vi "日期键盘.vi"(11 "原值":string) -> (3 "x+y":string)   [LabVIEW 2016]
uses:
  <vilib>/Utility/miscctls.llb/LVPointTypeDef.ctl
panel:
  in  "日":string(combo)="01"
  in  "月":string(combo)="01"
  in  "年":string(combo)="2000"
  in  "取消按钮":bool
  in  "停止":bool
  # "年"
  # "月"
  # "日"
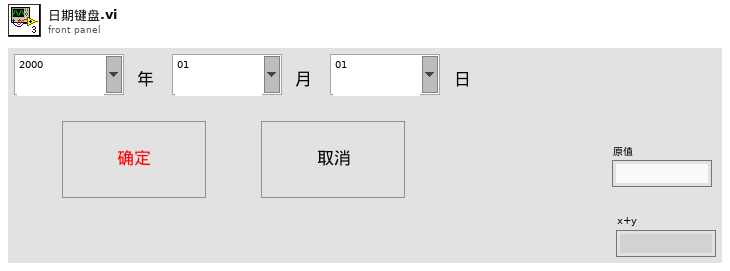
[diagram p1: front panel]
types:
  T1 = typedef "LVPointTypeDef.ctl" = cluster{"Horizontal":i16, "Vertical":i16}
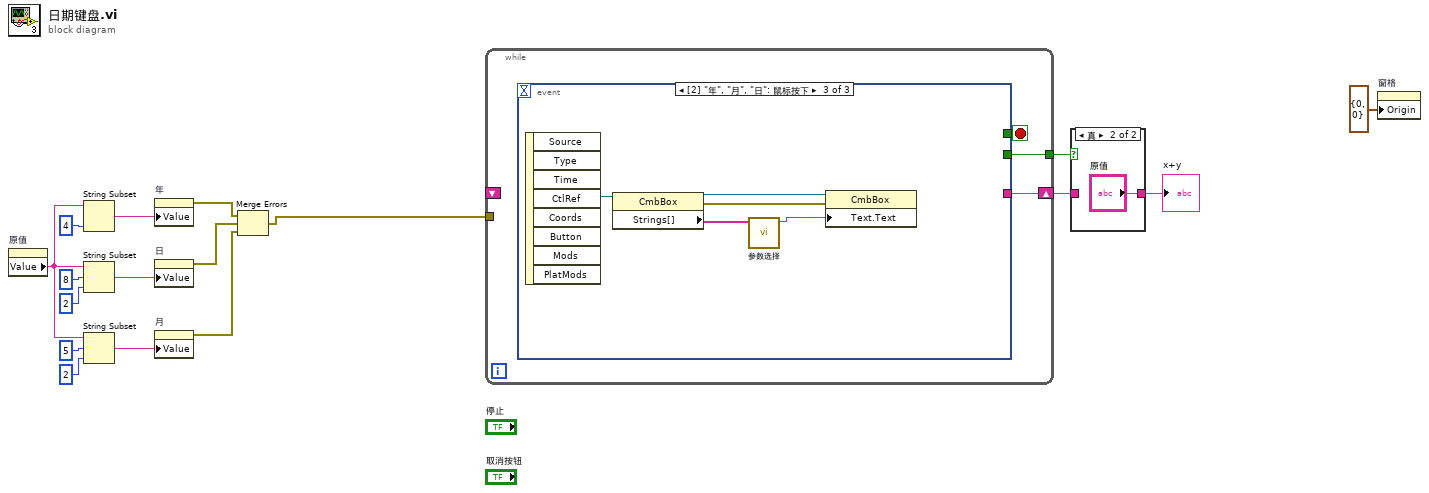
[diagram p0: block diagram]
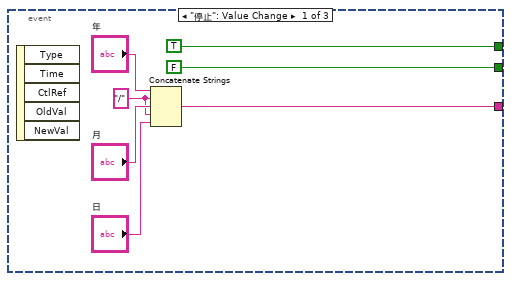
[diagram p3: hidden frame]
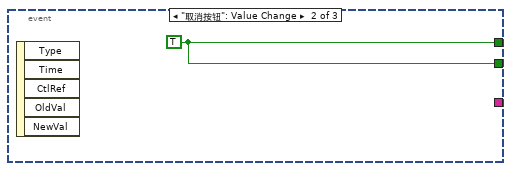
[diagram p4: hidden frame]
diagram:
  n1 = property on="原值" class="Str"() -> ("Value"=w9:string)  [unwired: 2 in, 2 out]
  n2 = String Subset(string=w9, length (rest)=4 ("长度（剩余）")) -> (substring=w12:string)  [unwired: 1 in]
  n3 = String Subset(string=w9, offset (0)=8 ("偏移量(0)"), length (rest)=2 ("长度（剩余）")) -> (substring=w5:string)
  n4 = String Subset(string=w9, offset (0)=5 ("偏移量(0)"), length (rest)=2 ("长度（剩余）")) -> (substring=w6:string)
  n5 = property on="年" class="CmbBox"("Value"=w12) -> (error out=w4:errorcluster)  [unwired: 2 in, 1 out]
  n6 = property on="日" class="CmbBox"("Value"=w5) -> (error out=w2:errorcluster)  [unwired: 2 in, 1 out]
  n7 = property on="月" class="CmbBox"("Value"=w6) -> (error out=w3:errorcluster)  [unwired: 2 in, 1 out]
  n8 = Merge Errors(w4, w2, w3) -> (w1:errorcluster)
  n9 = while {
    shift-right: [w18] -> w17
    shift-left: _ -> [_]
    tunnel: [w19] -> w15
    tunnel: w1 -> [_]
    stop <- w20 stop-if-true
    n10 = event shown="[2] \"年\", \"月\", \"日\": 鼠标按下" {
      selector: _ -> [_ _ _]
      dyn-events: _ -> [_ _ _]
      timeout: _ -> [_ _ _]
      tunnel: [TRUE w28 _] -> w20
      tunnel: [w21 _ _] -> w18
      tunnel: [FALSE w28 _] -> w19
      event "停止": Value Change {
        w22 = "/" ("字符串")
        n11 = event-data() -> ()  [unwired: 1 in, 5 out]
        n12 = Concatenate Strings("年", w22, "月", w22, "日") -> (w21:string)
      }
      event "取消按钮": Value Change {
        w28 = TRUE
        n13 = event-data() -> ()  [unwired: 1 in, 5 out]
      }
      event "年", "月", "日": Mouse Down {
        n14 = event-data() -> ("CtlRef"=w33:refnum<vi>)  [unwired: 1 in, 7 out]
        n15 = property class="CmbBox"(reference=w33) -> (reference out=w32:refnum<vi>, error out=w29:errorcluster, "Strings[]"=w31:string[])  [unwired: 1 in]
        n16 = call "参数选择.vi"("项名"=w31) -> ("字符串"=w30:string)  [unwired: 10 in]
        n17 = property class="CmbBox"(reference=w32, error in=w29, "Text.Text"=w30) -> ()  [unwired: 2 out]
      }
    }
  }
  n18 = case shown="真" w15 {
    tunnel: w17 -> [w34 _]
    tunnel: [w34 "原值"] -> w16
    frame False {
    }
    frame True {
    }
  }
  "x+y" <- w16
  n19 = property on="窗格" class="Pane"("Origin"=T1 {"Horizontal"=0, "Vertical"=0} ("原点")) -> ()  [unwired: 2 in, 2 out]
